vi "Coffee Timing (SubVI).vi"(7 "Function":enum16{"Reset Time", "Time Elapsed"}(ring), 8 "error in (no error)":errorcluster, 11 "Time to Wait (s)":i32) -> (0 "error out":errorcluster, 2 "Remaining Time":i32, 3 "Time elapsed ?":bool)   [LabVIEW 2017]
doc: "Dieses VI managt das Timing der Kaffeemaschine."
panel:
  # "Input Values"
  # "Output Values"
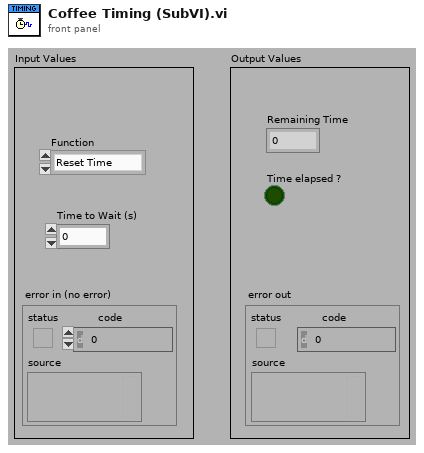
[diagram p1: front panel]
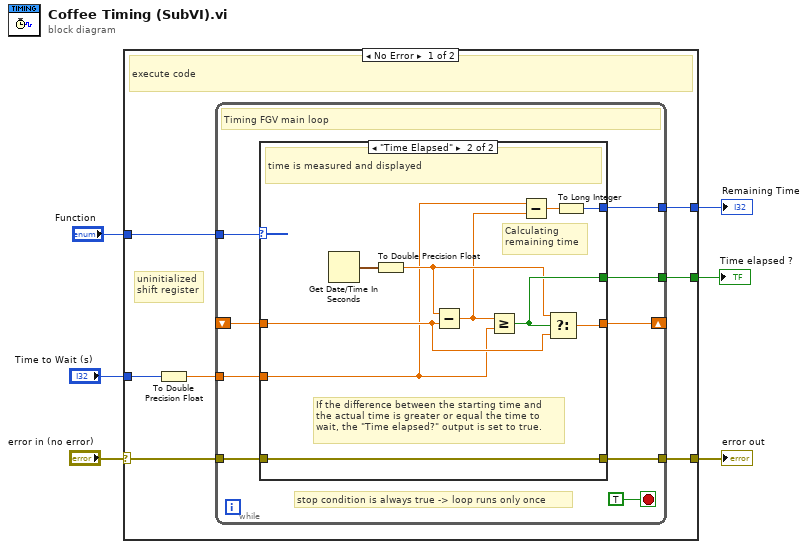
[diagram p0: block diagram]
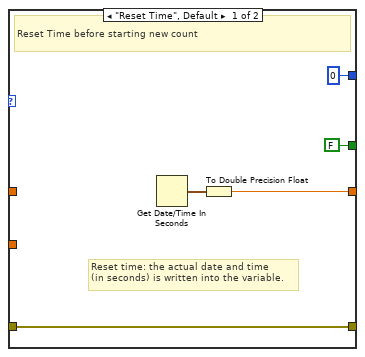
[diagram p2: hidden frame]
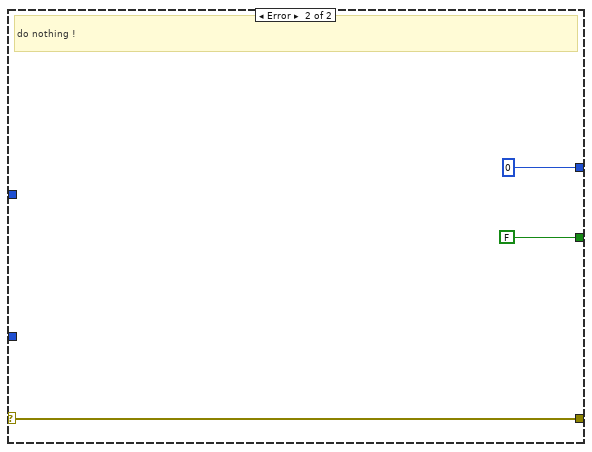
[diagram p3: hidden frame]
diagram:
  n1 = case shown="No Error" "error in (no error)" {
    selector: "error in (no error)" -> [w12 w40]
    tunnel: [w13 w40] -> w5
    tunnel: "Function" -> [w11 _]
    tunnel: "Time to Wait (s)" -> [w8 _]
    tunnel: [w10 FALSE] -> w3
    tunnel: [w9 0] -> w1
    frame No Error {
      # "uninitialized\nshift register"
      # "execute code"
      n2 = To Double Precision Float(number=w8) -> (double precision float=w7:dbl)
      n3 = while {
        shift-right: [w18] -> _
        shift-left: _ -> [w17]
        tunnel: [w21] -> w13
        tunnel: w12 -> [w20]
        tunnel: w11 -> [w19]
        tunnel: w7 -> [w16]
        tunnel: [w15] -> w10
        tunnel: [w14] -> w9
        stop <- TRUE stop-if-true
        # "stop condition is always true -> loop runs only once"
        # "Timing FGV main loop"
        n4 = case shown="\"Time Elapsed\"" w19 {
          tunnel: [w27 w37] -> w21
          tunnel: w20 -> [w27 w37]
          tunnel: [w25 w35] -> w18
          tunnel: w17 -> [_ w33]
          tunnel: w16 -> [_ w30]
          tunnel: [FALSE w34] -> w15
          tunnel: [0 w28] -> w14
          frame "Reset Time", Default {
            # "Reset time: the actual date and time \n(in seconds) is written into the variable."
            # "Reset Time before starting new count"
            n5 = Get Date/Time In Seconds() -> (seconds since 1Jan1904=w26:timestamp)
            n6 = To Double Precision Float(number=w26) -> (double precision float=w25:dbl)
          }
          frame "Time Elapsed" {
            # "Calculating\nremaining time"
            # "If the difference between the starting time and \nthe actual time is greater or equal the time to\nwait, the \"Time elapsed?\" output is set to true."
            # "time is measured and displayed"
            n7 = Get Date/Time In Seconds() -> (seconds since 1Jan1904=w36:timestamp)
            n8 = To Double Precision Float(number=w36) -> (double precision float=w32:dbl)
            n9 = Subtract(x=w32, y=w33) -> (x-y=w31:dbl)
            n10 = Greater Or Equal?(x=w31, y=w30) -> (x >= y?=w34:bool)
            n11 = Subtract(x=w30, y=w31) -> (x-y=w29:dbl)
            n12 = Select(t=w32, s=w34, f=w33) -> (s? t:f=w35:dbl)
            n13 = To Long Integer(number=w29) -> (32bit integer=w28:i32)
          }
        }
      }
    }
    frame Error {
      # "do nothing !"
    }
  }
  "error out" <- w5
  "Time elapsed ?" <- w3
  "Remaining Time" <- w1
